vi "TempMon2.vi"() -> ()   [LabVIEW 2011]
doc: "This VI will continuously monitor the serial port and extract the temperature reading from the received string. This is stored in an array and displayed on the Graph. Press STOP to close the serial port and end the program.\n\nThis program is designed to work with the May 2009 version of the Arduino Temperature program which sends a header, the raw A/D value and the temperature as a float text value.\n\nSelect the appropriate COM port before running this VI. Leave the other serial port settings at their default values (9600, 8, none, 1.0, none)."
uses:
  <vilib>/Instr/_visa.llb/VISA Configure Serial Port (Instr).vi
panel:
  out "concatenated string":string
  out "CurTemp":dbl caption="Current Temperature\n(Celsius)"
  in  "VISA resource name":refnum<visa-resource-name>="COM3"
  in  "baud rate (9600)":u32=9600
  in  "data bits (8)":u16=8 min=5 max=8 step=1
  in  "stop bits (10: 1 bit)":u16(ring)=10 items=["1.0"=10, "1.5"=15, "2.0"=20]
  in  "flow control (0:none)":u16(ring) items=["None", "XON/XOFF", "RTS/CTS", "XON/XOFF & RTS/CTS", "DTR/DSR", "XON/XOFF & DTR/DSR"]
  in  "parity (0:none)":enum16{"None", "Odd", "Even", "Mark", "Space"}(ring)
  in  "stop":bool
  out "TempArray":dbl[](array[numeric]) caption="Temperature Array"
  out "Temperature Graph":dbl[](graph)
  # "This VI will continuously monitor the serial port and extract the temperature reading from the received string.  This is stored in an array and displayed on the Graph.  Press STOP to close the serial port and end the program.\n\nThis program is designed to work with the March 2009 version of the Arduino Temperature program which sends a header, the raw A/D value and the temperature as an integer value.\n\nSelect the appropriate COM port before running this VI.  Leave the other serial port settings at their default values (9600, 8, none, 1.0, none)."
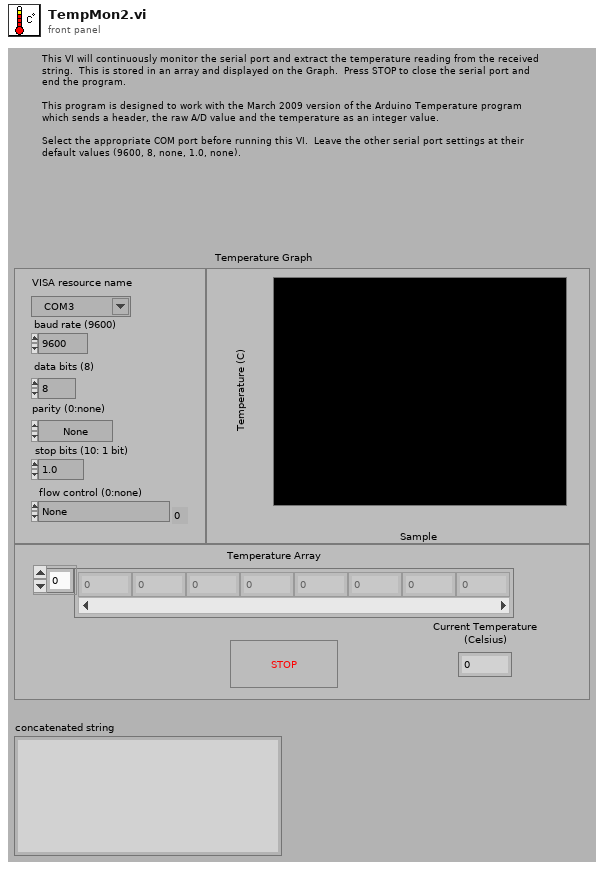
[diagram p1: front panel]
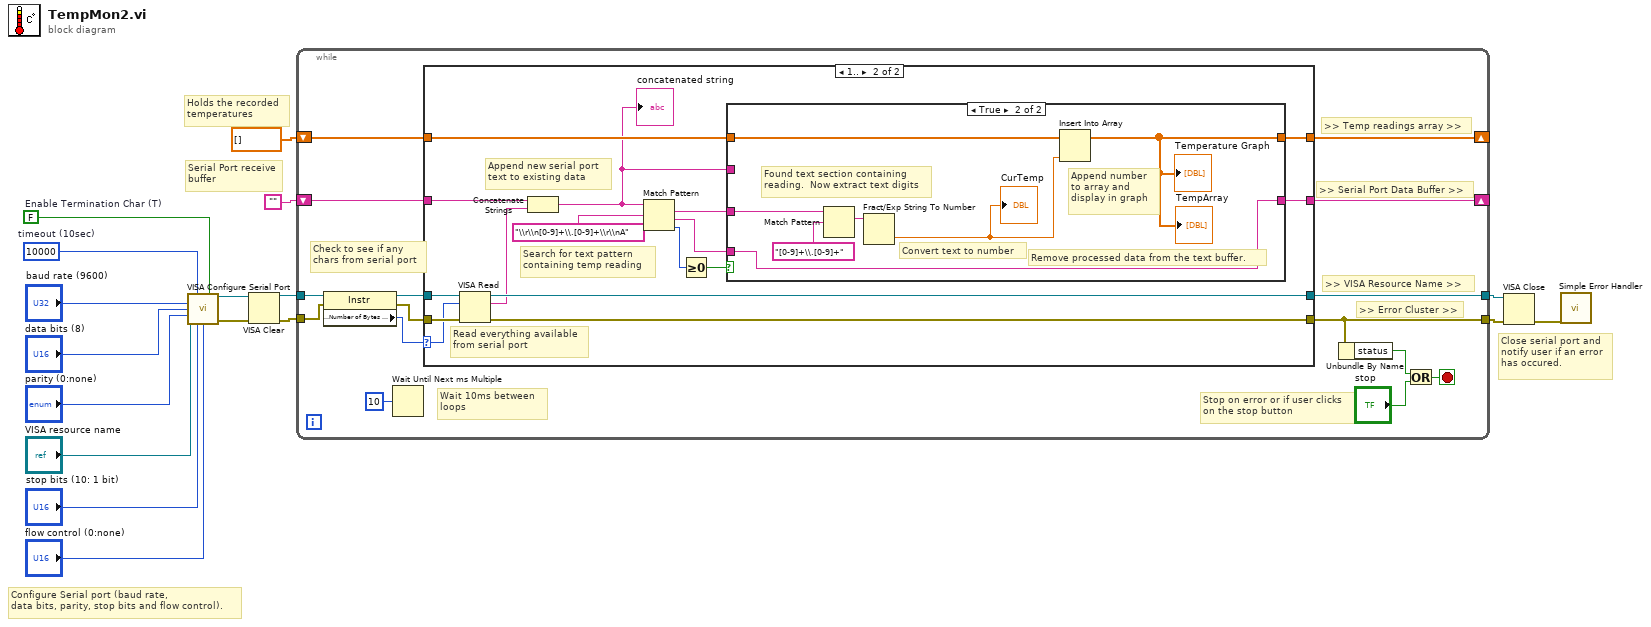
[diagram p0: block diagram]
diagram:
  w13 = FALSE  # Enable Termination Char (T)
  w14 = u32 10000  # timeout (10sec)
  # "Close serial port and\nnotify user if an error\nhas occured."
  # "Serial Port receive\nbuffer"
  # "Holds the recorded\ntemperatures"
  # "Configure Serial port (baud rate,\ndata bits, parity, stop bits and flow control)."
  n1 = call-poly "VISA Configure Serial Port"("VISA resource name"="VISA resource name", "timeout (10sec)"=w14, "Enable Termination\nChar (T)"=w13, "baud rate (9600)"="baud rate (9600)", "data bits (8)"="data bits (8)", "parity (0:none)"="parity (0:none)", "stop bits (10: 1 bit)"="stop bits (10: 1 bit)", "flow control (0:none)"="flow control (0:none)") -> ("VISA resource name out"=w11:refnum<visa-resource-name>, "error out"=w12:errorcluster)  [unwired: 6 in]
  n2 = VISA Clear(VISA resource name=w11, error in (no error)=w12) -> (VISA resource name out=w9:refnum<visa-resource-name>, error out=w8:errorcluster)
  n3 = while {
    tunnel: [w24] -> w17
    tunnel: [w32] -> w16
    shift-right: [w18] -> _
    shift-left: "" -> [w26]
    tunnel: w9 -> [w29]
    tunnel: w8 -> [w28]
    shift-right: [w20] -> _
    shift-left: dbl[] [] -> [w19]
    stop <- w23 stop-if-true
    # "Wait 10ms between \nloops"
    # "Stop on error or if user clicks \non the stop button"
    # ">> Error Cluster >>"
    # ">> VISA Resource Name >>"
    # ">> Temp readings array >>"
    # ">> Serial Port Data Buffer >>"
    # "Check to see if any\nchars from serial port"
    n4 = property class="Instr"(reference=w29, error in=w28) -> (reference out=w31:refnum<visa-resource-name>, error out=w30:errorcluster, "Serial Settings:Number of Bytes at Serial Port"=w27:u32)
    n5 = Wait Until Next ms Multiple(millisecond multiple=u32 10) -> ()  [unwired: 1 out]
    n6 = case shown="1.." w27 {
      selector: w27 -> [_ w46]
      tunnel: [w35 w52] -> w24
      tunnel: [w36 w51] -> w32
      tunnel: w31 -> [w36 w50]
      tunnel: w30 -> [w35 w49]
      tunnel: w26 -> [w34 w48]
      tunnel: [w34 w40] -> w18
      tunnel: [w33 w38] -> w20
      tunnel: w19 -> [w33 w39]
      frame 0, Default {
        # "No data in from serial port - Nothing to do."
      }
      frame 1.. {
        # "Search for text pattern\ncontaining temp reading"
        # "Append new serial port\ntext to existing data"
        # "Read everything available\nfrom serial port"
        n7 = VISA Read(VISA resource name=w50, byte count=w46, error in (no error)=w49) -> (VISA resource name out=w51:refnum<visa-resource-name>, read buffer=w47:string, error out=w52:errorcluster)  [unwired: 1 out]
        n8 = Concatenate Strings(w48, w47) -> (w37:string)
        "concatenated string" <- w37
        n9 = Match Pattern(string=w37, regular expression="\\r\\n[0-9]+\\.[0-9]+\\r\\nA") -> (match substring=w42:string, after substring=w41:string, offset past match=w44:i32)  [unwired: 1 in, 1 out]
        n10 = Greater Or Equal To 0?(x=w44) -> (x >= 0?=w43:bool)
        n11 = case shown="True" w43 {
          tunnel: w42 -> [_ w60]
          tunnel: w41 -> [_ w61]
          tunnel: w37 -> [w54 _]
          tunnel: [w54 w61] -> w40
          tunnel: [w53 w58] -> w38
          tunnel: w39 -> [w53 w57]
          frame False {
            # "Did not find text pattern in the buffer.  Try again in the next loop after new data \nhas been received."
          }
          frame True {
            # "Remove processed data from the text buffer."
            # "Append number\nto array and\ndisplay in graph"
            # "Convert text to number"
            # "Found text section containing \nreading.  Now extract text digits"
            n12 = Match Pattern(string=w60, regular expression="[0-9]+\\.[0-9]+") -> (match substring=w59:string)  [unwired: 1 in, 3 out]
            n13 = Fract/Exp String To Number(string=w59) -> (number=w55:dbl)  [unwired: 3 in, 1 out]
            "CurTemp" <- w55
            n14 = Insert Into Array(array=w57, new element=w55) -> (w58:dbl[])  [unwired: 1 in]
            "Temperature Graph" <- w58
            "TempArray" <- w58
          }
        }
      }
    }
    n15 = Unbundle By Name(w24) -> ("status"=w22:bool)
    n16 = Or(x=w22, y="stop") -> (x .or. y?=w23:bool)
  }
  n17 = VISA Close(VISA resource name=w16, error in (no error)=w17) -> (error out=w15:errorcluster)
  n18 = call <vilib>:"Simple Error Handler.vi"("error in (no error)"=w15) -> ()  [unwired: 4 in, 5 out]
